vi "Dither Right.vi"(5 "Label":string="Dither", 7 "Goal":T1, 8 "error in":errorcluster, 10 "Mask":string="Relative", 11 "Location":string=" ") -> (0 "error out":errorcluster, 3 "Location Out":string=" ")   [LabVIEW 2013]
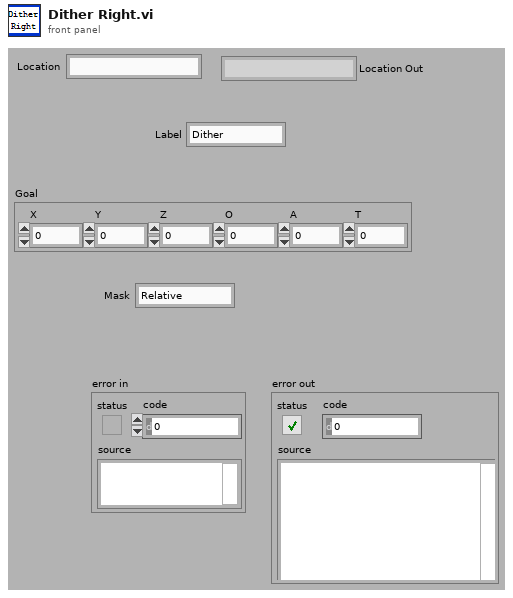
[diagram p1: front panel]
types:
  T1 = cluster{"X":dbl, "Y":dbl, "Z":dbl, "O":dbl, "A":dbl, "T":dbl}
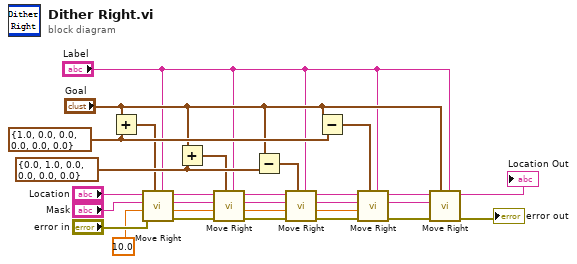
[diagram p0: block diagram]
diagram:
  w21 = T1 {"X"=0.0, "Y"=1.0, "Z"=0.0, "O"=0.0, "A"=0.0, "T"=0.0} ("Goal Axes")
  w1 = 10.0 ("Speed")
  w22 = T1 {"X"=1.0, "Y"=0.0, "Z"=0.0, "O"=0.0, "A"=0.0, "T"=0.0} ("Goal Axes")
  n1 = Add(x="Goal", y=w22) -> (x+y=w20:T1)
  n2 = call "Move Right.vi"("Label"="Label", "Goal"=w20, "error in"="error in", "Speed"=w1, "Mask"="Mask", "Location"="Location") -> ("error out"=w26:errorcluster, "Mask Out"=w9:string, "Location Out"=w14:string)  [unwired: 1 in, 2 out]
  n3 = Add(x="Goal", y=w21) -> (x+y=w19:T1)
  n4 = call "Move Right.vi"("Label"="Label", "Goal"=w19, "error in"=w26, "Speed"=w1, "Mask"=w9, "Location"=w14) -> ("error out"=w25:errorcluster, "Mask Out"=w8:string, "Location Out"=w13:string)  [unwired: 1 in, 2 out]
  n5 = Subtract(x="Goal", y=w21) -> (x-y=w18:T1)
  n6 = call "Move Right.vi"("Label"="Label", "Goal"=w18, "error in"=w25, "Speed"=w1, "Mask"=w8, "Location"=w13) -> ("error out"=w24:errorcluster, "Mask Out"=w7:string, "Location Out"=w12:string)  [unwired: 1 in, 2 out]
  n7 = Subtract(x="Goal", y=w22) -> (x-y=w16:T1)
  n8 = call "Move Right.vi"("Label"="Label", "Goal"=w16, "error in"=w24, "Speed"=w1, "Mask"=w7, "Location"=w12) -> ("error out"=w23:errorcluster, "Mask Out"=w6:string, "Location Out"=w11:string)  [unwired: 1 in, 2 out]
  n9 = call "Move Right.vi"("Label"="Label", "Goal"="Goal", "error in"=w23, "Mask"=w6, "Location"=w11) -> ("error out"=→"error out":errorcluster, "Location Out"=→"Location Out":string)  [unwired: 2 in, 3 out]
